vi "UI Build Listbox Items.vi"(8 "error in (no error)":errorcluster, 11 "GObject in":refnum<class "GObject.lvclass">) -> (0 "error out":errorcluster, 2 "GObject Item Strings (UTF-16)":string[][](array[string]), 3 "GObject out":refnum<class "GObject.lvclass">)   [LabVIEW 2013, in "SET Project Editor.lvlib" / "GObject View.lvclass"]
uses:
  GObject View.lvclass
  SET Project Data/Control Classes/GObject/GObject.lvclass
  SET Project Data/Control Classes/GObject/GObject.lvclass/GObject.ctl
  SET Project Data/Control Classes/GObject/Read Items.vi
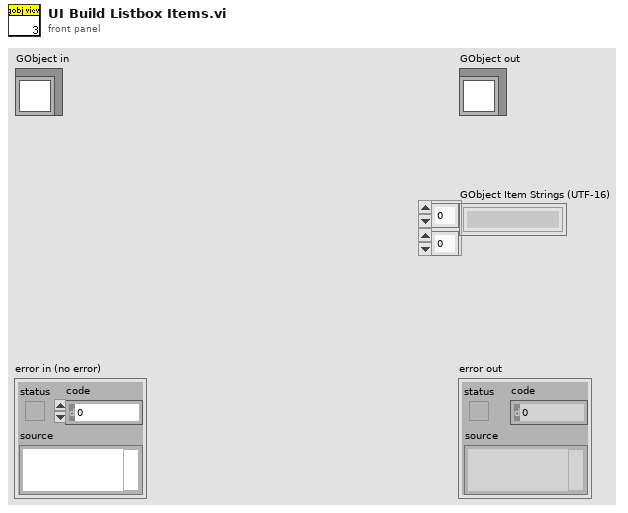
[diagram p1: front panel]
types:
  T1 = typedef "SET Project Data.lvlib/ProjFile_Resource Entry.ctl" = cluster{"RID":string, "Tag":string, "Strings [] (UTF-16)":string[], "Shared?":bool}
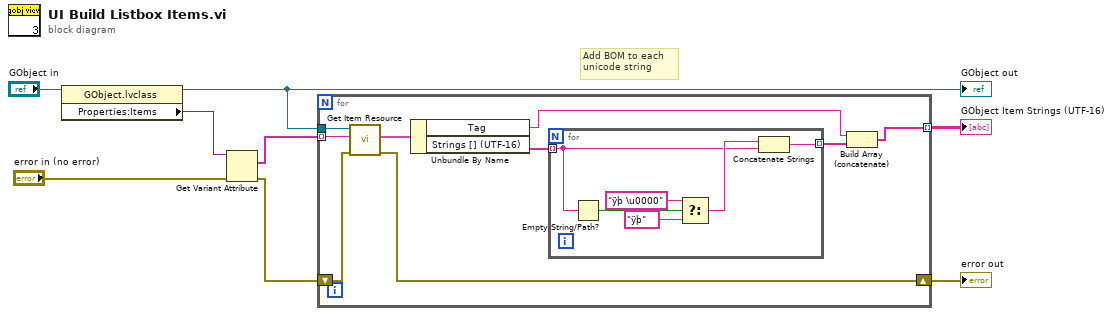
[diagram p0: block diagram]
diagram:
  # "Add BOM to each\nunicode string"
  n1 = property class="GObject.lvclass"(reference="GObject in") -> (reference out=w2:refnum<class "GObject.lvclass">, "Properties:Items"=w1:variant)  [unwired: 1 in, 1 out]
  "GObject out" <- w2
  n2 = Get Variant Attribute(Variant=w1, error in="error in (no error)") -> (names=w8:string[], error out=w5:errorcluster)  [unwired: 2 in, 2 out]
  n3 = for {
    tunnel: w2 -> [w17]
    tunnel: w8 -> [w16] mode=indexing
    shift-right: [w14] -> w4
    shift-left: w5 -> [w15]
    tunnel: [w9] -> w7 mode=indexing
    n4 = call "Get Item Resource.vi"("error in (no error)"=w15, "ItemName"=w16, "GObject in"=w17) -> ("error out"=w14:errorcluster, "Resource"=w13:T1)  [unwired: 4 in, 3 out]
    n5 = Unbundle By Name(w13) -> ("Tag"=w10:string, "Strings [] (UTF-16)"=w12:string[])
    n6 = for {
      tunnel: w12 -> [w19] mode=indexing
      tunnel: [w18] -> w11 mode=indexing
      n7 = Empty String/Path?(string/path=w19) -> (empty?=w23:bool)
      n8 = Select(t="ÿþ \u0000" ("string"), s=w23, f="ÿþ" ("string")) -> (s? t:f=w20:string)
      n9 = Concatenate Strings(w20, w19) -> (w18:string)
    }
    n10 = Build Array (concatenate)(w10, w11) -> (w9:string[])
  }
  "error out" <- w4
  "GObject Item Strings (UTF-16)" <- w7
